vi "get_pose_values.vi"(9 "First record":sgl[][](array[numeric]), 10 "Trace record":sgl[][](array[numeric]), 11 "Selector":T1) -> (3 "XYZ Rx Ry Rz":dbl[](array[numeric]))   [LabVIEW 2013]
uses:
  pose_selector.ctl
  pose_source.ctl
  pose_relative_to.ctl
  <vilib>/Analysis/coordinate.llb/Angle Units.ctl
  <vilib>/Analysis/baseanly.llb/Real A x B.vi
  <vilib>/Analysis/coordinate.llb/Wrap Angle (array).vi
  initialization/micron_globals.vi
  <vilib>/Analysis/Matrix/Numeric/Conversions/Array To Matrix - RA.vi
  <vilib>/Analysis/NI_AALBase.lvlib
  <vilib>/Analysis/Matrix/NI_Matrix.lvlib
  <vilib>/Analysis/NI_AAL_Angle.lvlib
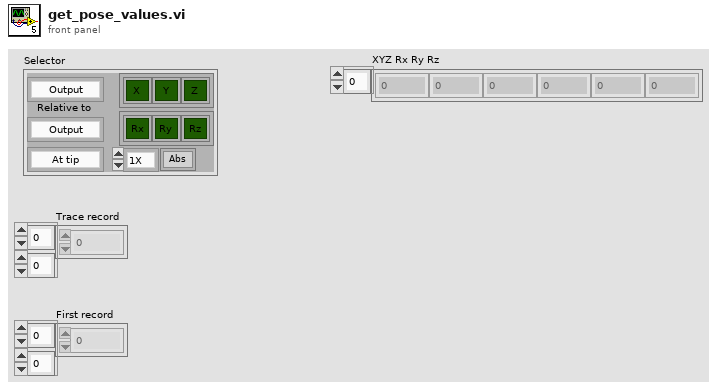
[diagram p1: front panel]
types:
  T1 = typedef "pose_selector.ctl" = cluster{"Scale":enum16{"1X", "10X", "100X", "1KX", "10KX"}, "Source":T2, "XYZ selector":cluster{"Boolean":bool, "Boolean 2":bool, "Boolean 3":bool}, "RPY selector":cluster{"Boolean":bool, "Boolean 2":bool, "Boolean 3":bool}, "Relative to":T3, "Relative":bool, "Translate":enum16{"At tip", "At RCM", "At KC", "At origin"}}
  T2 = typedef "pose_source.ctl" = enum16{"Output", "Handle", "Handle KF", "Goal", "Absolute"}
  T3 = typedef "pose_relative_to.ctl" = enum16{"Output", "Handle", "Handle KF", "Goal", "Absolute", "Trace start"}
  T4 = typedef "NI_AAL_Angle.lvlib/Angle Units.ctl" = i32
  T5 = typedef "Micron params.ctl" = cluster{"Stimulus":T6, "Goal Filter A":T8, "Mode controls":T9, "Manipulator type":enum16{"Current piezo", "Voltage piezo"}, "Manipulator calibration":T10, "Network":T12, "Goal Filter B":T8, "Cancellation":T13, "Transition time":sgl, "Estimation":T15}
  T6 = typedef "stimulus.ctl" = cluster{"Type":enum16{"Off", "Step", "Sine", "Triangle", "Arbitrary"}, "Phase":dbl, "Amplitude":sgl[], "Injection point":T7, "Closed loop":bool, "Offset":sgl[], "Tip -> world":bool, "Frequency":dbl, "Length":dbl}
  T7 = typedef "injection_point.ctl" = enum16{"Total pose", "V limiter", "Goal ", "Link position", "KF link position", "Inverse kin", "Link goal", "Link error", "Controller", "Output", "Drive", "Light"}
  T8 = typedef "goal_loop_parms.ctl" = cluster{"Speedup max":sgl, "Speedup thresh":sgl, "Speedup nonlin":sgl, "Filters":cluster{"Lower Fc":sgl, "Lower Q":sgl, "Scale factor":sgl, "Upper Fc":sgl, "Upper Q":sgl, "V limit":sgl, "V limit range":sgl}[]}
  T9 = typedef "mode_conrols.ctl" = cluster{"Hold":bool, "Cancellation":bool, "Goal filter":bool, "Trigger":bool}
  T10 = typedef "manipulator_cal.ctl" = cluster{"Tool offsets":sgl[][], "Tip light calibration":T11, "Handle light calibration":T11, "Base pivots":sgl[][], "Output pivots":sgl[][], "Length center":sgl, "Workspace height":sgl[], "Workspace diameter":sgl[], "Linearization":sgl[][], "Stack travel":sgl, "Saturation pos":sgl, "Inverse filters":cluster{"filter structure":enum32{"IIR 2nd Order", "IIR 4th Order"}, "Reverse Coefficients":dbl[], "Forward Coefficients":dbl[]}[]}
  T11 = typedef "probe_calibration.ctl" = sgl[][]
  T12 = typedef "network_params.ctl" = cluster{"Remote Host":string, "Send Status":bool, "Send Port":u16, "Recv Commands":bool, "Recv Port":u16}
  T13 = typedef "sq_control_params.ctl" = cluster{"KP":T14, "KI":sgl, "KD":T14, "Max vel":sgl, "Max acc":sgl, "Int error limit":sgl, "RCM gain":sgl, "Bypass":bool, "Degraded gain":sgl}
  T14 = typedef "decoupled_gain.ctl" = cluster{"XY":sgl, "Rxy":sgl, "Z":sgl, "Rz":sgl}
  T15 = typedef "estimation_controls.ctl" = cluster{"Link":cluster{"Measure noise":dbl[], "Process noise":dbl[], "Alt process noise":dbl[], "Alt turnoff cycles":i32, "Innovation limit":dbl[], "Residue threshold":dbl, "Enable":bool}, "Handle":cluster{"Measure noise":dbl[], "Process noise":dbl[], "State limits":dbl[], "Innovation limit":dbl[], "Prediction Lookahead":sgl, "Enable":bool}}
  T16 = typedef "NI_Matrix.lvlib/RealMatrix.ctl" = dbl[][]
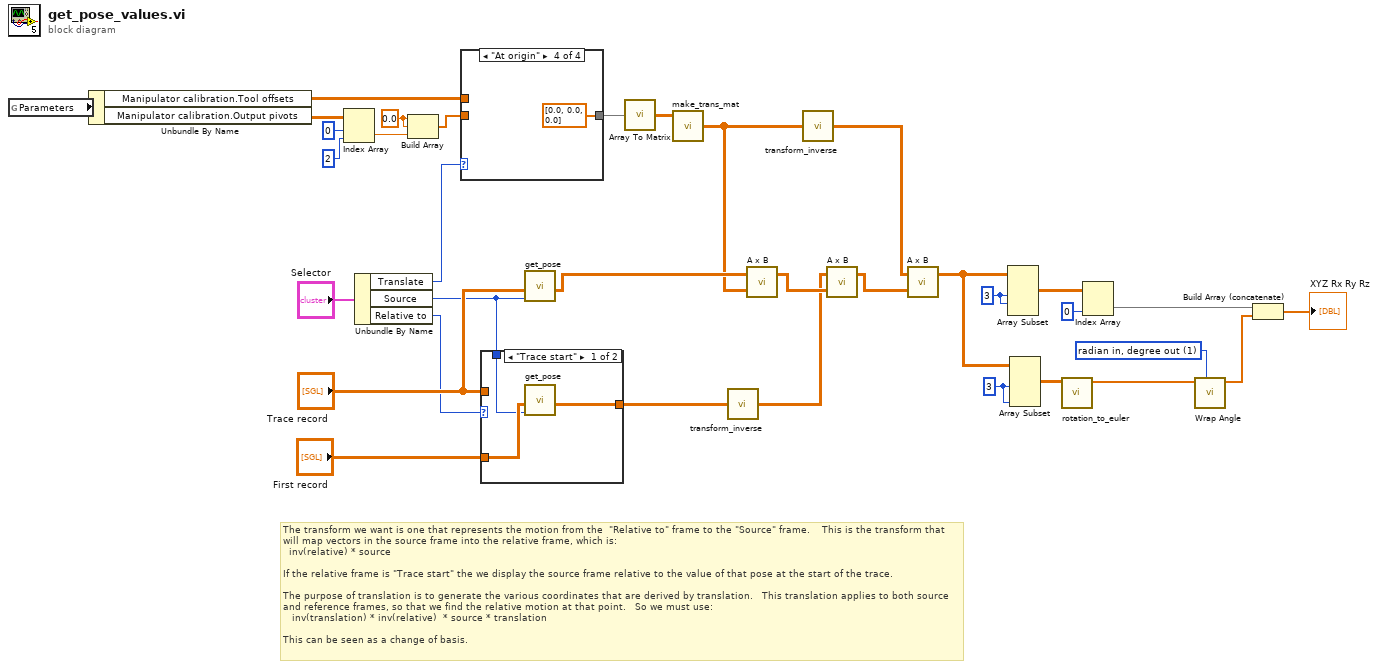
[diagram p0: block diagram]
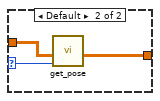
[diagram p2: hidden frame]
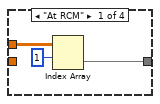
[diagram p3: hidden frame]
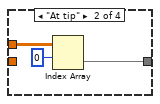
[diagram p4: hidden frame]
diagram:
  w4 = T4 1 items=["radian in, radian out", "radian in, degree out", "degree in, degree out", "degree in, radian out"] ("angle units")
  w18 = sgl 0.0 ("element")
  w29 = 3 ("length")
  w31 = 3 ("length")
  # "The transform we want is one that represents the motion from the  \"Relative to\" frame to the \"Source\" frame.    This is the transform that will map vectors in the source frame into the relative frame, which is:\n  inv(relative) * source\n\nIf the relative frame is \"Trace start\" the we display the source frame relative to the value of that pose at the start of the trace.\n\nThe purpose of translation is to generate the various coordinates that are derived by translation.   This translation applies to both source and reference frames, so that we find the relative motion at that point.   So we must use:\n   inv(translation) * inv(relative)  * source * translation\n\nThis can be seen as a change of basis."
  n1 = global read "micron_globals.vi" "Parameters"() -> (w23:T5)
  n2 = Unbundle By Name(w23) -> ("Manipulator calibration.Tool offsets"=w17:sgl[][], "Manipulator calibration.Output pivots"=w22:sgl[][])
  n3 = Index Array(array=w22, index (row)=0 ("disabled index (row)"), index (col)=2 ("disabled index (col)")) -> (element=w19:sgl)
  n4 = Unbundle By Name("Selector") -> ("Translate"=w24:enum16{"At tip", "At RCM", "At KC", "At origin"}, "Source"=w1:T2, "Relative to"=w3:T3)
  n5 = Build Array(w18, w18, w19) -> (w16:sgl[])
  n6 = case shown="\"At origin\"" w24 {
    tunnel: w17 -> [w37 w40 _ _]
    tunnel: [w35 w38 w41 sgl[] [0.0, 0.0, 0.0] ("Tool offsets")] -> w13
    tunnel: w16 -> [_ _ w41 _]
    frame "At RCM" {
      n7 = Index Array(array=w37, index (row)=1) -> (element=w35:sgl[])  [unwired: 1 in]
    }
    frame "At tip" {
      n8 = Index Array(array=w40, index (row)=0) -> (element=w38:sgl[])  [unwired: 1 in]
    }
    frame "At KC" {
    }
    frame "At origin" {
    }
  }
  n9 = case shown="\"Trace start\"" w3 {
    selector: w3 -> [_ w46]
    tunnel: [w45 w48] -> w34
    tunnel: "Trace record" -> [_ w47]
    tunnel: "First record" -> [w44 _]
    tunnel: w1 -> [w43 _]
    frame "Trace start" {
      n10 = call "get_pose.vi"("Selector"=w43, "Input Trace"=w44) -> ("Pose"=w45:T16)  [unwired: 9 in]
    }
    frame Default {
      n11 = call "get_pose.vi"("Selector"=w46, "Input Trace"=w47) -> ("Pose"=w48:T16)  [unwired: 9 in]
    }
  }
  n12 = call "get_pose.vi"("Selector"=w1, "Input Trace"="Trace record") -> ("Pose"=w14:T16)  [unwired: 9 in]
  n13 = call-poly <vilib>:"Array To Matrix.vi"("Real 1D Array"=w13) -> ("Real Matrix (Column Vector)"=w15:T16)
  n14 = call "make_trans_mat.vi"("Translation"=w15) -> ("Transform"=w10:T16)  [unwired: 4 in]
  n15 = call "transform_inverse.vi"("Transform"=w34) -> ("Inverse transform"=w11:T16)
  n16 = call-poly <vilib>:"A x B.vi"("B"=w10, "A"=w14) -> ("A x B"=w12:T16)  [unwired: 1 out]
  n17 = call "transform_inverse.vi"("Transform"=w10) -> ("Inverse transform"=w8:T16)
  n18 = call-poly <vilib>:"A x B.vi"("B"=w12, "A"=w11) -> ("A x B"=w9:T16)  [unwired: 1 out]
  n19 = call-poly <vilib>:"A x B.vi"("B"=w9, "A"=w8) -> ("A x B"=w7:T16)  [unwired: 1 out]
  n20 = Array Subset(array=w7, length (row)=w29, index (col)=w29) -> (w27:T16)  [unwired: 2 in]
  n21 = Array Subset(array=w7, length (row)=w31, length (col)=w31) -> (w30:T16)  [unwired: 2 in]
  n22 = call "rotation_to_euler.vi"("Rotation"=w30) -> ("Theta XYZ"=w6:dbl[])  [unwired: 10 in]
  n23 = Index Array(array=w27, index (col)=0 ("disabled index (col)")) -> (element=w25:dbl[])  [unwired: 1 in]
  n24 = call-poly <vilib>:"Wrap Angle.vi"("angle units"=w4, "Angle In"=w6) -> ("Angle Out"=w5:dbl[])  [unwired: 8 in, 1 out]
  n25 = Build Array (concatenate)(w25, w5) -> (→"XYZ Rx Ry Rz":dbl[])
